vi "Serial Number.vi"(8 "error in (no error)":errorcluster, 11 "EPU452 in":refnum<class "EPU452.lvclass">) -> (0 "error out":errorcluster, 2 "Serial Number":string, 3 "EPU452 out":refnum<class "EPU452.lvclass">)   [LabVIEW 2018, in "EPU452.lvclass"]
uses:
  EPU452.lvclass
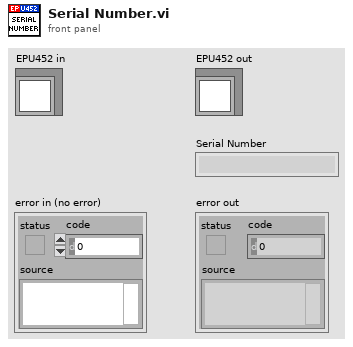
[diagram p1: front panel]
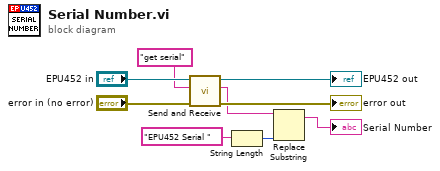
[diagram p0: block diagram]
diagram:
  n1 = call "Send and Receive.vi"("error in (no error)"="error in (no error)", "Command"="get serial", "EPU452 in"="EPU452 in") -> ("error out"=→"error out":errorcluster, "Response"=w3:string, "EPU452 out"=→"EPU452 out":refnum<class "EPU452.lvclass">)  [unwired: 6 in]
  n2 = String Length(string="EPU452 Serial ") -> (length=w1:i32)
  n3 = Replace Substring(2:w1, 5:w3) -> (1:→"Serial Number":string)  [unwired: 2 in, 1 out]
